vi "GetResistanceProperties.vi"(11 "Properties":T1[](array[typedef])) -> (3 "Range Mode":u32)   [LabVIEW 2017, in "ScanEngine.lvlib"]
uses:
  <vilib>/addons/InsightCM/Devices/Shared/Common/ScanEngine/ScanEngine.lvlib
  <vilib>/addons/InsightCM/MessageBus/Base/controls/KeyValuePair.ctl
  <vilib>/addons/InsightCM/Utilities/PropertyHelpers/PropertyHelpers.lvlib
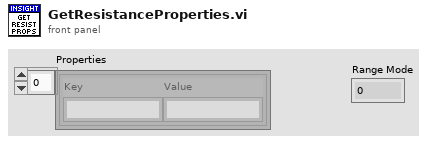
[diagram p1: front panel]
types:
  T1 = typedef "KeyValuePair.ctl" = cluster{"Key":string, "Value":string}
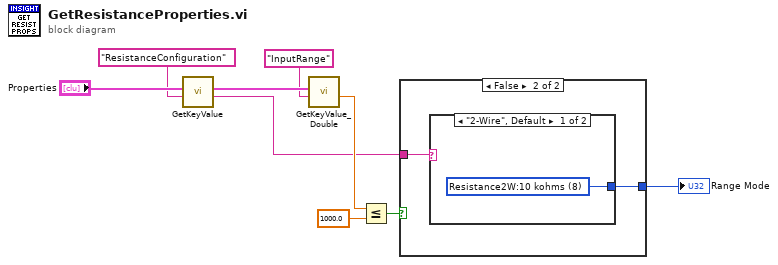
[diagram p0: block diagram]
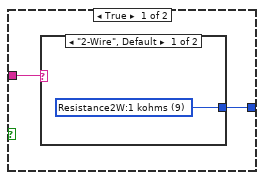
[diagram p2: hidden frame]
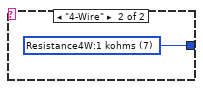
[diagram p3: hidden frame]
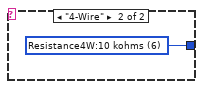
[diagram p4: hidden frame]
diagram:
  n1 = call <vilib>:"GetKeyValue.vi"("key"="ResistanceConfiguration" ("name"), "key value pairs"="Properties") -> ("value"=w1:string, "key value pairs out"=w5:T1[])  [unwired: 7 in, 1 out]
  n2 = call <vilib>:"GetKeyValue_Double.vi"("key"="InputRange" ("name"), "key value pairs"=w5) -> ("value"=w3:dbl)  [unwired: 7 in, 2 out]
  n3 = Less Or Equal?(x=w3, y=1000.0) -> (x <= y?=w8:bool)
  n4 = case shown="False" w8 {
    tunnel: w1 -> [w10 w15]
    tunnel: [w11 w14] -> w7
    frame True {
      n5 = case shown="\"2-Wire\", Default" w10 {
        tunnel: [w12 w13] -> w11
        frame "2-Wire", Default {
          w12 = u32 9 items=["Voltage:60 V", "Voltage:15 V", "Voltage:4 V", "Voltage:1 V", "Voltage:125 mV", "Current:25 mA", "Resistance4W:10 kohms", "Resistance4W:1 kohms", "Resistance2W:10 kohms", "Resistance2W:1 kohms", "Thermocouple", "RTD4W:Pt1000", "RTD4W:Pt100", "RTD3W:Pt1000", "RTD3W:Pt100", "QuarterBridge:350 ohm", "QuarterBridge:120 ohm", "HalfBridge:500 mV/V", "FullBridge:625 mV/V", "FullBridge:78 mV/V", "DigitalIn", "OpenContact"] ("9129 Mode")
        }
        frame "4-Wire" {
          w13 = u32 7 items=["Voltage:60 V", "Voltage:15 V", "Voltage:4 V", "Voltage:1 V", "Voltage:125 mV", "Current:25 mA", "Resistance4W:10 kohms", "Resistance4W:1 kohms", "Resistance2W:10 kohms", "Resistance2W:1 kohms", "Thermocouple", "RTD4W:Pt1000", "RTD4W:Pt100", "RTD3W:Pt1000", "RTD3W:Pt100", "QuarterBridge:350 ohm", "QuarterBridge:120 ohm", "HalfBridge:500 mV/V", "FullBridge:625 mV/V", "FullBridge:78 mV/V", "DigitalIn", "OpenContact"] ("9129 Mode")
        }
      }
    }
    frame False {
      n6 = case shown="\"2-Wire\", Default" w15 {
        tunnel: [w16 w17] -> w14
        frame "2-Wire", Default {
          w16 = u32 8 items=["Voltage:60 V", "Voltage:15 V", "Voltage:4 V", "Voltage:1 V", "Voltage:125 mV", "Current:25 mA", "Resistance4W:10 kohms", "Resistance4W:1 kohms", "Resistance2W:10 kohms", "Resistance2W:1 kohms", "Thermocouple", "RTD4W:Pt1000", "RTD4W:Pt100", "RTD3W:Pt1000", "RTD3W:Pt100", "QuarterBridge:350 ohm", "QuarterBridge:120 ohm", "HalfBridge:500 mV/V", "FullBridge:625 mV/V", "FullBridge:78 mV/V", "DigitalIn", "OpenContact"] ("9129 Mode")
        }
        frame "4-Wire" {
          w17 = u32 6 items=["Voltage:60 V", "Voltage:15 V", "Voltage:4 V", "Voltage:1 V", "Voltage:125 mV", "Current:25 mA", "Resistance4W:10 kohms", "Resistance4W:1 kohms", "Resistance2W:10 kohms", "Resistance2W:1 kohms", "Thermocouple", "RTD4W:Pt1000", "RTD4W:Pt100", "RTD3W:Pt1000", "RTD3W:Pt100", "QuarterBridge:350 ohm", "QuarterBridge:120 ohm", "HalfBridge:500 mV/V", "FullBridge:625 mV/V", "FullBridge:78 mV/V", "DigitalIn", "OpenContact"] ("9129 Mode")
        }
      }
    }
  }
  "Range Mode" <- w7
